vi "traceFileIO_writeToFile.vi"(0 "reference in":refnum<class "OSA.lvclass">, 1 "Path":path, 2 "file format (SPF2)":T2(ring)=enum."SPF2", 3 "dataType":T3, 4 "trace idx":u32, 5 "error in (no error)":errorcluster, 7 "dialog (empty path)":bool) -> (13 "global trace idx":u32, 14 "reference out":refnum<class "OSA.lvclass">, 15 "actual path":path, 17 "cancelled":bool, 19 "error out":errorcluster)   [LabVIEW 2010, in "OSA.lvclass"]
doc: "Read spectrum or interferogram data from a trace buffer, (FTSLib.dll allocated), and write to file."
uses:
  OSA.lvclass
  typeDef/acq_dataType.ctl
  typeDef/trace_properties_ui.ctl
  FTSLib.dll
  OSA20X_misc.lvlib
panel:
  in  "property":T1
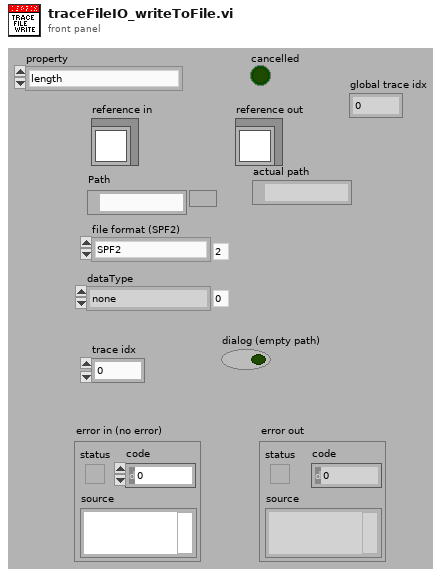
[diagram p1: front panel]
types:
  T1 = typedef "OSA.lvclass/trace_properties_ui.ctl" = enum16{"length", "type", "acquisitionMode", "xValueFormat", "date", "time", "averageNum", "smoothType", "igramSmoothType", "phaseCorrection", "apodisation", "__allocatedLengthI", "__allocatedLengthx", "adcBits", "sensitivityMode", "resolutionMode", "rollingAverage", "samplesPerReference", "air_measureOption", "interferogramProperty", "all_uiProperties"}
  T2 = enum16{"SPC", "CSV", "SPF2", "TXT", "MAT_V5", "CSV_ZIP", "TXT_ZIP", "JCAMPDX"}
  T3 = typedef "OSA.lvclass/acq_dataType.ctl" = enum16{"none", "interferogram", "spectrum"}
  T4 = typedef "OSA.lvclass/ObjectAttributes.ctl" = cluster{"Stop":bool, "dataType":T3, "spectrometerIdx":u16, "buffer size interferogram":i32, "interferogram":cluster{"new":bool, "plot_x_ min":sgl, "plot_x_max":sgl, "plot_y_min":sgl, "plot_y_max":sgl, "Graph Intrfrgrm":T5, "timeStamp":u32, "signal (%)":dbl, "traces":cluster{"idx":u32, "broadBand":bool, "monoChromatic":bool, "peakToPeakSignal":dbl, "peakToPeakPos":dbl}[], "traces idx last":i32}, "spectrum":cluster{"new":bool, "plot_x_min":sgl, "plot_x_max":sgl, "plot_unit_x":T6, "plot_unit_y":T7, "plot_y_min":sgl, "plot_y_max":sgl, "Graph Spectrum":T5, "timeStamp":u32, "X_VAL_OPTIONS":enum16{"MIN_MAX", "ARRAY"}, "traces":cluster{"idx":u32}[], "traces idx last":i32}, "Thorlabs_OSA_64.lvclass:queue_action.ctlqueue ref":refnum<queue>, "action":T8, "plot zoom step":dbl, "buffer semaphore":T9, "acq stopped":bool, "dataType active":T3, "temperature (degr C)":sgl, "pressure (hPa)":sgl, "rel humidity (%)":sgl, "settings":cluster{"resolution":u16, "sensitivity":u16, "Average":bool, "average nr":u32, "apodisation":T10, "acq delay (ms)":u32, "airMesure":T11, "wmtr on":bool, "intfgrm_smooth_width":u16, "intfgrm_smooth_nrOfPasses":u16, "intfgrm_smooth":T12, "phaseCorrection":T13, "zeroFill":u8, "spectr_smooth":T12, "spectr_smooth_width":u16, "spectr_smooth_nrOfPasses":u16, "resolution (/cm)":sgl, "REF wavelength, (nm)":dbl, "gain_idx":u16, "gainAuto":bool, "gain_relative":dbl, "PD sensitivity mode":T14, "PD senseMode implemented":bool, "SensorTemperature implemented":bool, "SensorPressure implemented":bool, "SensorHumidity implemented":bool}, "peaks position":sgl[], "peaks width":sgl[], "peaks height":sgl[], "peaks max nr":u32, "peaks latest nr":i32, "peaks new":bool, "power":dbl, "power new":bool, "path":string, "wavelength (WNr)":dbl, "wavelength new":bool, "buffer size spectrum":i32, "status":string, "VI reference":refnum<vi>, "funcPointer":u64, "libraryPointer":u64, "singleAcquisition":bool, "coherenceLength (cm)":dbl, "coherenceLength new":bool, "spectrometer model":string, "spectrometer serial nr":string, "peaks thld left":sgl[], "peaks thld right":sgl[], "coherenceLength error (cm)":dbl, "ADC bits":u16, "peaks position centroid":sgl[], "peaks height centroid":sgl[], "OSA series":T15, "channel index spectrum":u16, "spectrometer rangeLow, (/cm)":dbl, "spectrometer rangeHigh, (/cm)":dbl, "channel index interferogram":u16}
  T5 = typedef "OSA.lvclass/graph_intensity.ctl" = refnum<vi>
  T6 = typedef "OSA.lvclass/spectrum_x_unit.ctl" = enum16{"wavenr/cm", "THz", "eV", "nm_air", "nm_vac"}
  T7 = typedef "OSA.lvclass/y_unit.ctl" = enum16{"ADC counts", "dBm pwr absolute", "dBm pwr density", "mW pwr absolute", "mW pwr density"}
  T8 = typedef "OSA.lvclass/queue_action.ctl" = enum16{"none", "stop", "GUI_plotInterferogram", "GUI_plotSpectrum", "GUI_plotInterferogramRescale", "GUI_plotSpectrumRescale", "GUI_plotInterferogramReset", "GUI_plotSpectrumReset", "GUI_plotInterferogramAutoScaleY", "GUI_plotSpectrumAutoScaleY", "GUI_plotInterferogramZoomOut", "GUI_plotSpectrumZoomOut", "GUI_plotInterferogramPane", "GUI_plotSpectrumPane", "GUI_plotInterferogramZoomMouse", "GUI_plotSpectrumZoomMouse", "ENVIRONMENT temperature", "ENVIRONMENT pressure", "MODE_resolution set", "MODE_resolution get", "MODE_sensitivity set", "MODE_sensitivity get", "MODE_PDTemperature set", "MODE_PDTemperature get", "REBOOT/RESET firmware", "ACQASYNC_acquireSingleSpectrum", "ACQASYNC_continuous start", "ACQASYNC_continuous stop\n", "ACQASYNC_get last interferogram", "ACQASYNC_get last spectrum", "ACQASYNC_get last waveNr", "ACQOPT_interferogram smoothing set", "ACQOPT_interferogram smoothing get", "ACQOPT_spectrum smoothing set", "ACQOPT_spectrum smoothing get", "ACQOPT_apodisation type set", "ACQOPT_apodisation type get", "ACQOPT_phase correction type set", "ACQOPT_phase correction type get", "ACQOPT_acqIntervall_set", "ACQOPT_acqIntervall_get", "ACQOPT_average spectrum set", "ACQOPT_average spectrum get", "ACQOPT_rolling average set", "ACQOPT_rolling average get", "ACQOPT_zero fill factor set", "ACQOPT_zero fill factor get", "ACQOPT_cycle counting set", "ACQOPT_cycle counting get", "ACQOPT_air measure option set", "ACQOPT_air measure option get", "ACQOPT_gainLevel auto get", "ACQOPT_gainLevel auto set", "ACQOPT_gainLevel get", "ACQOPT_gainLevel set", "ACQOPT_getAll", "INSTRUMENT_PROPERTY_range_WaveNr_min", "INSTRUMENT_PROPERTY_range_WaveNr_max", "INSTRUMENT_PROPERTY_reference_wavelength_cm^-1", "INSTRUMENT_PROPERTY_samplesPerRefPeriod", "INSTRUMENT_PROPERTY_resolution_waveNrPercm", "INSTRUMENT_PROPERTY_availableGainLevels", "INSTRUMENT_PROPERTY_status", "CONVERT", "ANALYSE_POWER", "ANALYSE_PEAKS", "ANALYSE_WAVELENGTH", "ANALYSE_SPECTRUM", "ANALYSE_INTERFEROGRAM", "ANALYSE_COHERENCE_LENGTH", "MATH", "MATH_power", "MATH_peaks", "FILE", "miscellaneous"}
  T9 = typedef "Semaphore RefNum" = refnum<k1>
  T10 = typedef "OSA.lvclass/apodisation.ctl" = enum16{"NONE", "NORTON_BEER_WEAK", "NORTON_BEER_MEDIUM", "NORTON_BEER_STRONG", "TRIANGULAR", "COSINE", "HANN", "HAMMING", "BLACKMANHARRIS3", "BLACKMANHARRIS4", "GAUSSIAN"}
  T11 = typedef "OSA.lvclass/airMeasure.ctl" = enum16{"TEMPERATURE", "PRESSURE"}
  T12 = typedef "OSA20X_misc.lvlib/interferogram_smoothing.ctl" = enum16{"NONE", "BINOMIAL", "SAVITSKY_GOLAY", "FOURIER", "MOVING_AVERAGE", "GAUSSIAN"}
  T13 = typedef "OSA.lvclass/phaseCorrection.ctl" = enum16{"NONE", "MERTZ", "FORMAN", "MERTZ_FILE", "FORMAN_FILE", "FUTURE COMP."}
  T14 = typedef "OSA20X_misc.lvlib/PDTemperatureMode.ctl" = enum16{"cool: better sensitivity/noise floor", "warm: extended wl range"}
  T15 = typedef "OSA.lvclass/OSA_series.ctl" = enum16{"OSA200", "OSA300", "UNKNOWN"}
  T16 = cluster{"idx":u32, "broadBand":bool, "monoChromatic":bool, "peakToPeakSignal":dbl, "peakToPeakPos":dbl}[]
  T17 = cluster{"property":string, "property value":u32}[]
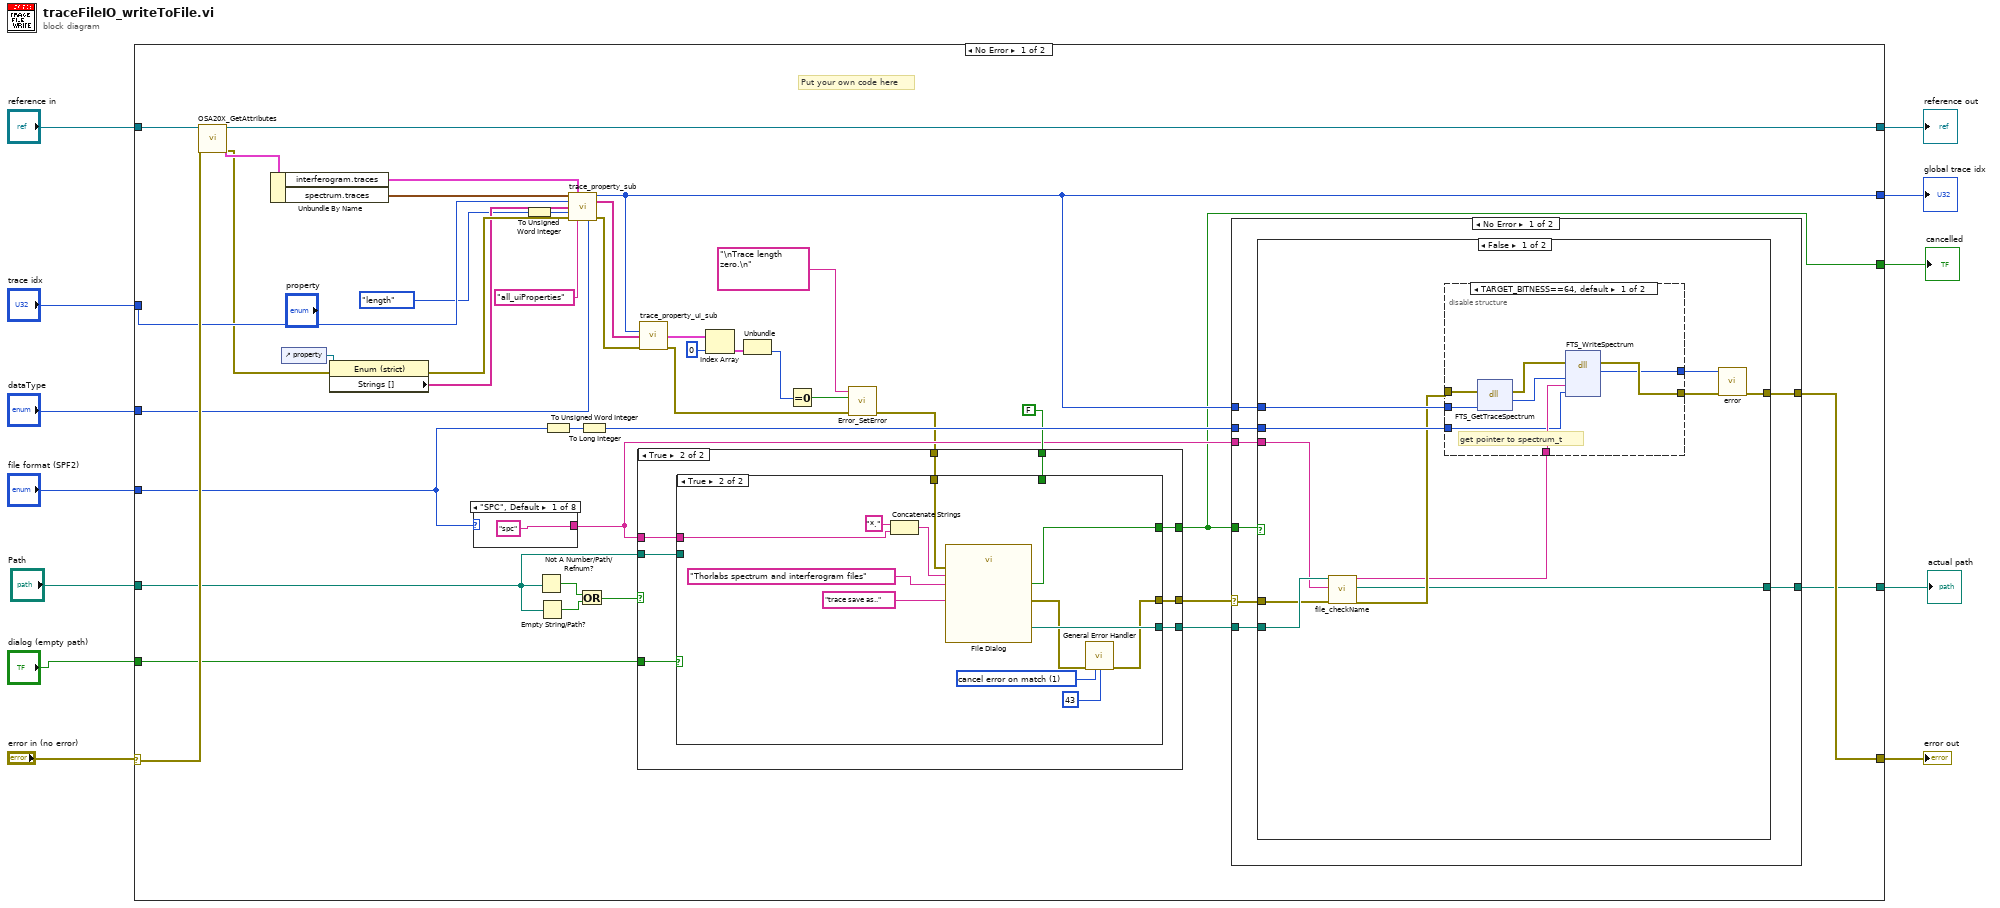
[diagram p0: block diagram]
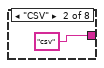
[diagram p2: hidden frame]
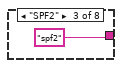
[diagram p3: hidden frame]
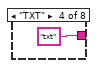
[diagram p4: hidden frame]
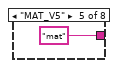
[diagram p5: hidden frame]
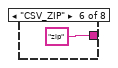
[diagram p6: hidden frame]
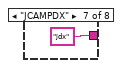
[diagram p7: hidden frame]
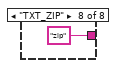
[diagram p8: hidden frame]
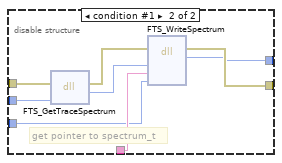
[diagram p9: hidden frame]
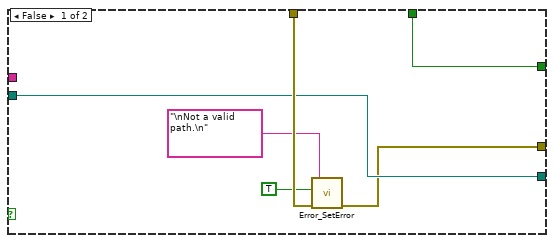
[diagram p13: hidden frame]
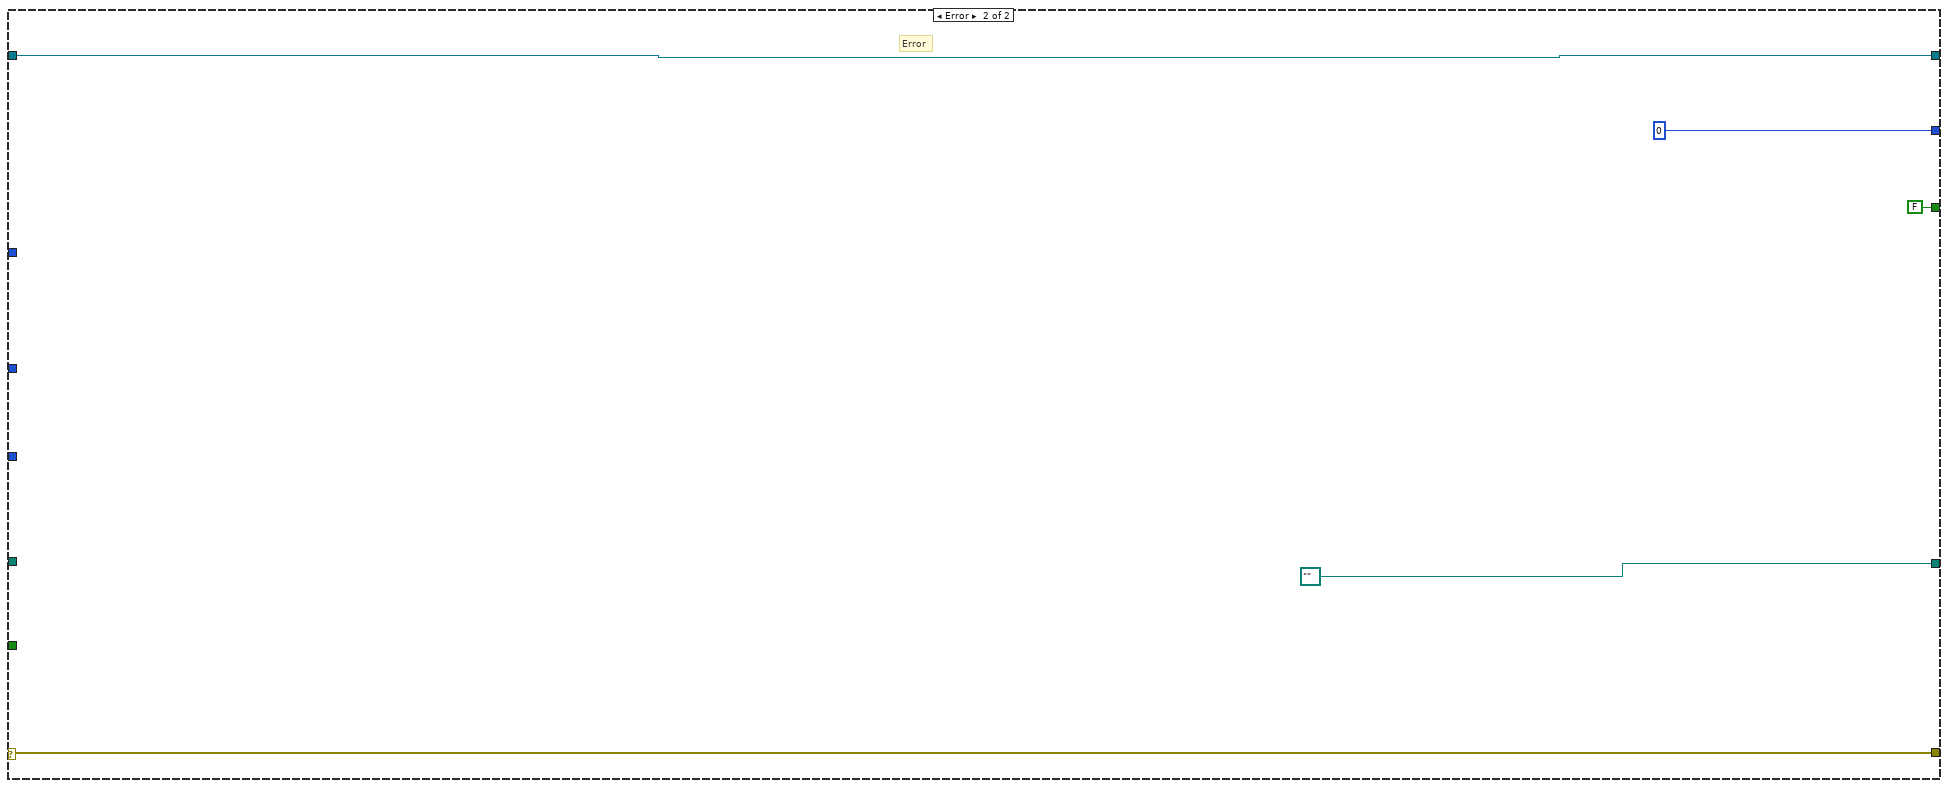
[diagram p14: hidden frame]
diagram:
  n1 = case shown="No Error" "error in (no error)" {
    selector: "error in (no error)" -> [w52 w134]
    tunnel: [w45 w134] -> w12
    tunnel: "reference in" -> [w51 w133]
    tunnel: [w50 w133] -> w9
    tunnel: "dataType" -> [w28 _]
    tunnel: "trace idx" -> [w29 _]
    tunnel: [w30 u32 0 ("global trace idx")] -> w6
    tunnel: "Path" -> [w46 _]
    tunnel: "dialog (empty path)" -> [w44 _]
    tunnel: "file format (SPF2)" -> [w38 _]
    tunnel: [w36 path "" ("selected path")] -> w2
    tunnel: [w13 FALSE ("cancelled")] -> w1
    frame No Error {
      # "Put your own code here"
      n2 = call "OSA20X_GetAttributes.vi"("reference in"=w51, "error in (no error)"=w52) -> ("reference out"=w50:refnum<class "OSA.lvclass">, "Data"=w53:T4, "error out"=w23:errorcluster)  [unwired: 14 in, 1 out]
      n3 = Unbundle By Name(w53) -> ("interferogram.traces"=w26:T16, "spectrum.traces"=w27:cluster{"idx":u32}[])
      n4 = control-ref of="property"() -> (w24:refnum<vi>)
      n5 = property class="Enum (strict)"(reference=w24, error in=w23) -> (error out=w22:errorcluster, "Strings []"=w21:string[])  [unwired: 1 out]
      n6 = case shown="\"SPC\", Default" w38 {
        tunnel: ["spc" "csv" "spf2" ("pattern (all files)") "txt" ("pattern (all files)") "mat" ("pattern (all files)") "zip" ("pattern (all files)") "jdx" ("pattern (all files)") "zip" ("pattern (all files)")] -> w37
        frame "SPC", Default {
        }
        frame "CSV" {
        }
        frame "SPF2" {
        }
        frame "TXT" {
        }
        frame "MAT_V5" {
        }
        frame "CSV_ZIP" {
        }
        frame "JCAMPDX" {
        }
        frame "TXT_ZIP" {
        }
      }
      n7 = To Unsigned Word Integer(number=trace_properties_ui."length" ("property")) -> (unsigned 16bit integer=w31:u16)
      n8 = Not A Number/Path/Refnum?(number/path/refnum=w46) -> (NaN/Path/Refnum?=w48:bool)
      n9 = Empty String/Path?(string/path=w46) -> (empty?=w49:bool)
      n10 = To Unsigned Word Integer(number=w38) -> (unsigned 16bit integer=w41:u16)
      n11 = call "trace_property_sub.vi"("traces_spectrum"=w27, "traces_interferogram"=w26, "trace idx"=w29, "Strings enum"=w21, "Value enum"=w31, "error in (no error)"=w22, "all string"="all_uiProperties", "dataType"=w28) -> ("global trace idx"=w30:u32, "parameter names"=w34:string[], "error out"=w25:errorcluster)  [unwired: 4 in, 1 out]
      n12 = Or(x=w48, y=w49) -> (x .or. y?=w47:bool)
      n13 = To Long Integer(number=w41) -> (32bit integer=w40:i32)
      n14 = call "trace_property_ui_sub.vi"("trace idx global"=w30, "properties ui"=w34, "error in (no error)"=w25) -> ("properties"=w35:T17, "error out"=w15:errorcluster)  [unwired: 10 in, 1 out]
      n15 = Index Array(array=w35, index=0) -> (element=w18:cluster{"property":string, "property value":u32})
      n16 = Unbundle(w18) -> ("property value"=w17:u32)  [unwired: 1 out]
      n17 = Equal To 0?(x=w17) -> (x = 0?=w16:bool)
      n18 = call "Error_SetError.vi"("error in"=w15, "status (true)"=w16, "source(\"\")"="\nTrace length zero.\n" ("source(\"\")")) -> ("error out"=w14:errorcluster)  [unwired: 4 in]
      n19 = case shown="True" w47 {
        tunnel: w46 -> [w102 w107]
        tunnel: w44 -> [_ w111]
        tunnel: w14 -> [w103 w110]
        tunnel: [w101 w108] -> w13
        tunnel: [w102 w109] -> w42
        tunnel: [w103 w106] -> w43
        tunnel: FALSE ("cancelled") -> [w101 w105]
        tunnel: w37 -> [_ w104]
        frame False {
        }
        frame True {
          n20 = case shown="True" w111 {
            tunnel: w110 -> [w117 w127]
            tunnel: [w114 w126] -> w109
            tunnel: [w112 w125] -> w108
            tunnel: w107 -> [w114 _]
            tunnel: [w113 w119] -> w106
            tunnel: w105 -> [w112 _]
            tunnel: w104 -> [_ w118]
            frame False {
              n21 = call "Error_SetError.vi"("error in"=w117, "status (true)"=TRUE, "source(\"\")"="\nNot a valid path.\n" ("source(\"\")")) -> ("error out"=w113:errorcluster)  [unwired: 4 in]
            }
            frame True {
              w122 = 1 items=["no exception", "cancel error on match", "set error on match"] ("[exception action] (none:0)")
              n22 = Concatenate Strings("*." ("string"), w118) -> (w123:string)
              n23 = call "File Dialog"("prompt"="trace save as..", "error in"=w127, "pattern (all files)"=w123, "pattern label"="Thorlabs spectrum and interferogram files") -> ("selected path"=w126:path, "cancelled"=w125:bool, "error out"=w120:errorcluster)  [unwired: 8 in, 1 out]
              n24 = call <vilib>:"General Error Handler.vi"("error in (no error)"=w120, "[exception action] (none:0)"=w122, "[exception code]"=43) -> ("error out"=w119:errorcluster)  [unwired: 8 in, 4 out]
            }
          }
        }
      }
      n25 = case shown="No Error" w43 {
        selector: w43 -> [w65 w100]
        tunnel: w30 -> [w69 _]
        tunnel: [w68 w100] -> w45
        tunnel: w13 -> [w64 _]
        tunnel: w42 -> [w67 w99]
        tunnel: w40 -> [w66 _]
        tunnel: w37 -> [w63 _]
        tunnel: [w62 w99] -> w36
        frame No Error {
          n26 = case shown="False" w64 {
            tunnel: w69 -> [w80 _]
            tunnel: [w79 w98] -> w68
            tunnel: w67 -> [w75 w97]
            tunnel: w66 -> [w78 _]
            tunnel: w65 -> [w74 w98]
            tunnel: w63 -> [w73 _]
            tunnel: [w70 w97] -> w62
            frame False {
              n27 = call "file_checkName.vi"("path"=w75, "filename extension"=w73, "error in (no error)"=w74) -> ("path string out"=w71:string, "actual path"=w70:path, "error out"=w72:errorcluster)  [unwired: 13 in, 1 out]
              n28 = disable-structure shown="TARGET_BITNESS==64, default" {
                disable-tunnel: w80 -> [w88 w93]
                disable-tunnel: w71 -> [w87 w92]
                disable-tunnel: w72 -> [w84 w94]
                disable-tunnel: [w83 w91] -> w77
                disable-tunnel: [w82 w90] -> w76
                disable-tunnel: w78 -> [w81 w89]
                frame condition #0 (active) {
                  # "get pointer to spectrum_t"
                  n29 = dll-call lib="FTSLib.dll" fn="FTS_GetTraceSpectrum"(error in=w84, "traceIdx"=w88) -> (error out=w85:errorcluster, "spectrum_t_pointer"=w86:u64)  [unwired: 3 in, 1 out]
                  n30 = dll-call lib="FTSLib.dll" fn="FTS_WriteSpectrum"(error in=w85, "spectrum_t_pointer"=w86, "fileNameAndPath"=w87, "fileFormat"=w81) -> (error out=w83:errorcluster, "returnValue"=w82:u32)  [unwired: 5 in, 1 out]
                }
                frame condition #1 {
                  # "get pointer to spectrum_t"
                  n31 = dll-call lib="FTSLib.dll" fn="FTS_GetTraceSpectrum"(error in=w94, "traceIdx"=w93) -> (error out=w95:errorcluster, "spectrum_t_pointer"=w96:u32)  [unwired: 3 in, 1 out]
                  n32 = dll-call lib="FTSLib.dll" fn="FTS_WriteSpectrum"(error in=w95, "spectrum_t_pointer"=w96, "fileNameAndPath"=w92, "format"=w89) -> (error out=w91:errorcluster, "parameter"=w90:u32)  [unwired: 5 in, 1 out]
                }
              }
              n33 = call "error.vi"("result code"=w76, "error in (no error)"=w77) -> ("error out"=w79:errorcluster)  [unwired: 15 in, 2 out]
            }
            frame True {
            }
          }
        }
        frame Error {
        }
      }
    }
    frame Error {
      # "Error"
    }
  }
  "error out" <- w12
  "reference out" <- w9
  "global trace idx" <- w6
  "actual path" <- w2
  "cancelled" <- w1
